vi "Aero_Tunnel_Server.vi"() -> ()   [LabVIEW 2011]
uses:
  Controls/Launch_controls/Aero_Tunnel_Server.ctl
panel:
  in  "stop":bool
  in  "reference":T1
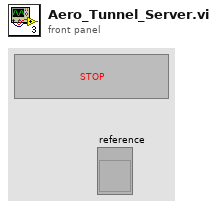
[diagram p1: front panel]
types:
  T1 = typedef "Aero_Tunnel_Server.ctl" = refnum<vi>
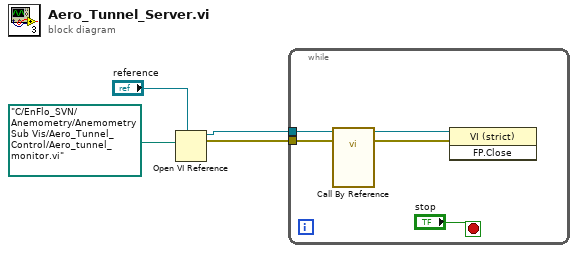
[diagram p0: block diagram]
diagram:
  n1 = Open VI Reference(type specifier VI Refnum (for type only)="reference", vi path=path "C:/EnFlo_SVN/Anemometry/Anemometry Sub Vis/Aero_Tunnel_Control/Aero_tunnel_monitor.vi") -> (vi reference=w2:T1, error out=w1:errorcluster)  [unwired: 4 in]
  n2 = while {
    tunnel: w2 -> [w9]
    tunnel: w1 -> [w8]
    stop <- "stop" stop-if-true
    n3 = call-by-ref "?"(reference=w9, error in=w8) -> (reference out=w5:T1, error out=w6:errorcluster)  [unwired: 1 in]
    n4 = invoke class="VI (strict)" method="FP.Close"(reference=w5, error in=w6) -> ()  [unwired: 1 in, 3 out]
  }
